vi "Deviated Result.vi"(8 "Error in":errorcluster, 11 "Data Converter in":refnum<class "Data Converter.lvclass">) -> (0 "Error out":errorcluster, 3 "Data Converter out":refnum<class "Data Converter.lvclass">)   [LabVIEW 2020]
doc: "Dynamic method to calculate deviated result"
uses:
  Data Converter.lvclass
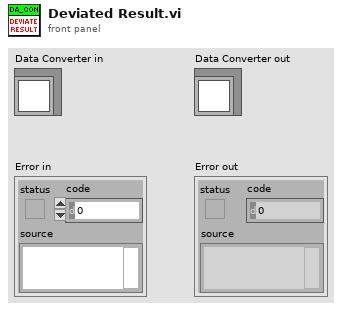
[diagram p1: front panel]
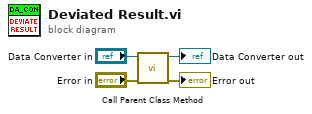
[diagram p0: block diagram]
diagram:
  n1 = call-parent "Call Parent Class Method"("Error in"="Error in", "Device in"="Data Converter in") -> ("Error out"=→"Error out":errorcluster, "Device out"=→"Data Converter out":refnum<class "Data Converter.lvclass">)  [unwired: 8 in]
